vi "Case.vi"(8 "error in (no error)":errorcluster, 10 "ShiftR":refnum<class "ShiftR.lvclass">, 11 "Abstract in":refnum<class "Abstract.lvclass">) -> (0 "error out":errorcluster, 1 "Exit":bool, 2 "ShiftR out":refnum<class "ShiftR.lvclass">, 3 "Abstract out":refnum<class "Abstract.lvclass">)   [LabVIEW 2021, in "Msn Trasnsportation Library 1.lvlib" / "Abstract.lvclass"]
uses:
  Abstract.lvclass
  ShiftR/ShiftR.lvclass
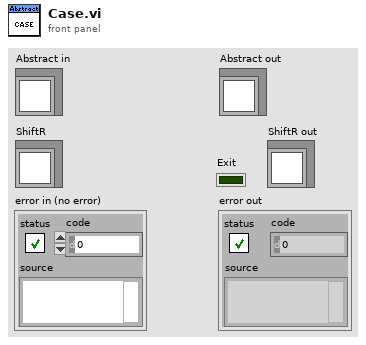
[diagram p1: front panel]
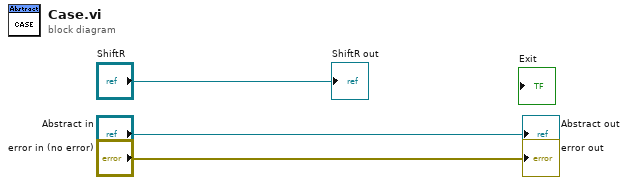
[diagram p0: block diagram]
diagram:
  "error out" <- "error in (no error)"
  "Abstract out" <- "Abstract in"
  "ShiftR out" <- "ShiftR"
